vi "Parse GULP Output file.vi"(10 "Reference Energy/atom (pure Crystal) (eV/atom)":dbl=-3.17454527875, 11 "GULP output file":path) -> (0 "Total Lattice Energy (eV)":dbl, 1 "Interfacial Energy (mJ/m²)":dbl, 2 "GB DoF":dbl[](array[numeric]), 3 "Final Structure":T1, 4 "# of atoms":i32, 5 "Data":string[](array[string]))   [LabVIEW 2010]
uses:
  <vilib>/Analysis/NI_AALPro.lvlib
panel:
  out "Lattice vector c":dbl[](array[numeric])
  out "Lattice vector b":dbl[](array[numeric])
  out "Lattice vector a":dbl[](array[numeric])
  out "Grain Boundary Definition":T2={"Grain 1 Orientation"=[1.0, 1.0, 1.0], "Grain 2 Orientation"=[1.0, 1.0, 1.0], "Twist Angle (Deg)"=60.0, "Translation Vector"=[0.0, 0.0, 0.0]}
  out "Headers":string[](array[string])
  out "Initial Structure":T1
  out "GB Area":dbl
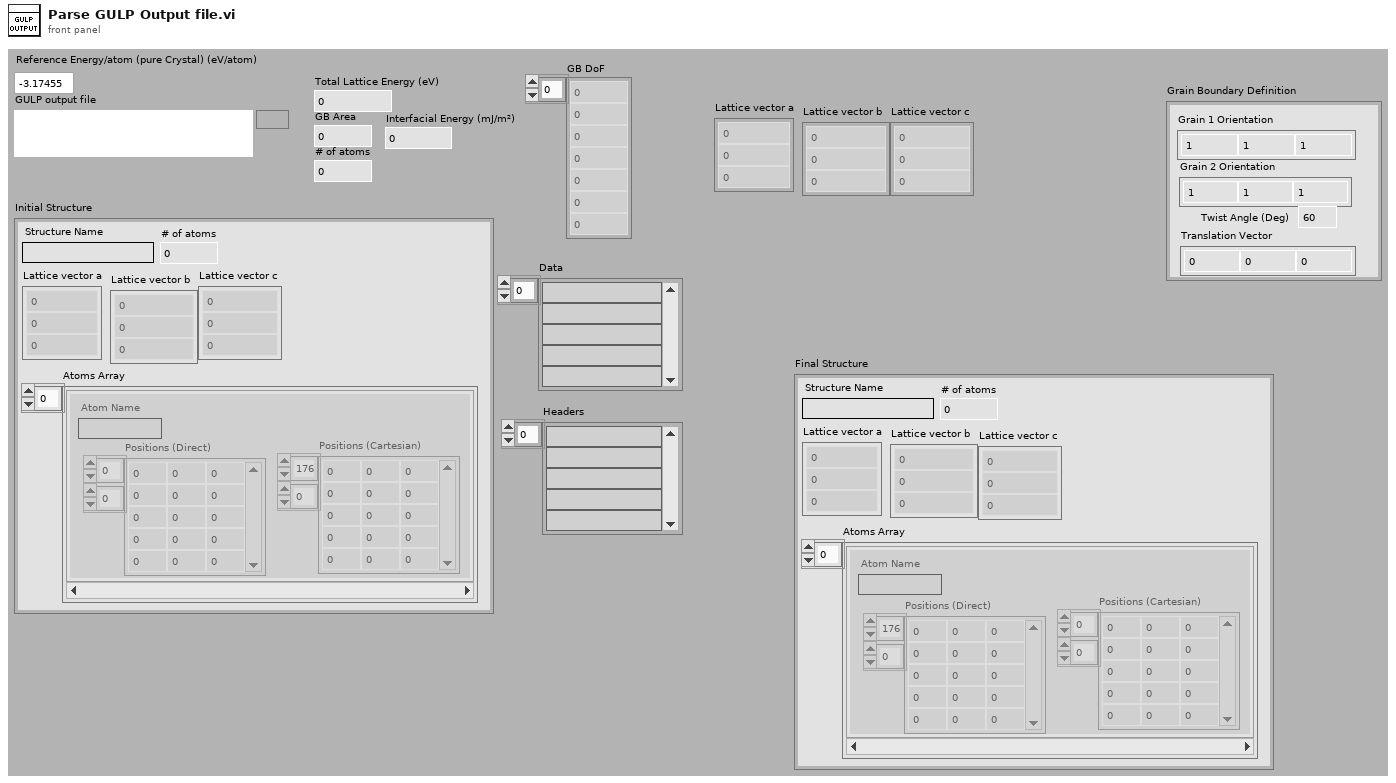
[diagram p1: front panel]
types:
  T1 = cluster{"Structure Name":string, "Lattice vector a":dbl[], "Lattice vector b":dbl[], "Lattice vector c":dbl[], "Atoms Array":cluster{"Atom Name":string, "Positions (Direct)":dbl[][], "Positions (Cartesian)":dbl[][]}[], "# of atoms":i32}
  T2 = cluster{"Grain 1 Orientation":dbl[], "Grain 2 Orientation":dbl[], "Twist Angle (Deg)":dbl, "Translation Vector":dbl[]}
  T3 = cluster{"Atom Name":string, "Positions (Direct)":dbl[][]}[]
  T4 = cluster{"Atom Name":string, "Positions (Direct)":dbl[][]}
  T5 = cluster{"token string":string, "Positions (Direct)":dbl[][]}[]
  T6 = cluster{"Atom Name":string, "Positions (Direct)":dbl[][], dbl[][]}
  T7 = cluster{string, "Lattice vector a":dbl[], "Lattice vector b":dbl[], "Lattice vector c":dbl[], cluster{"Atom Name":string, "Positions (Direct)":dbl[][], dbl[][]}[], "# of atoms":i32}
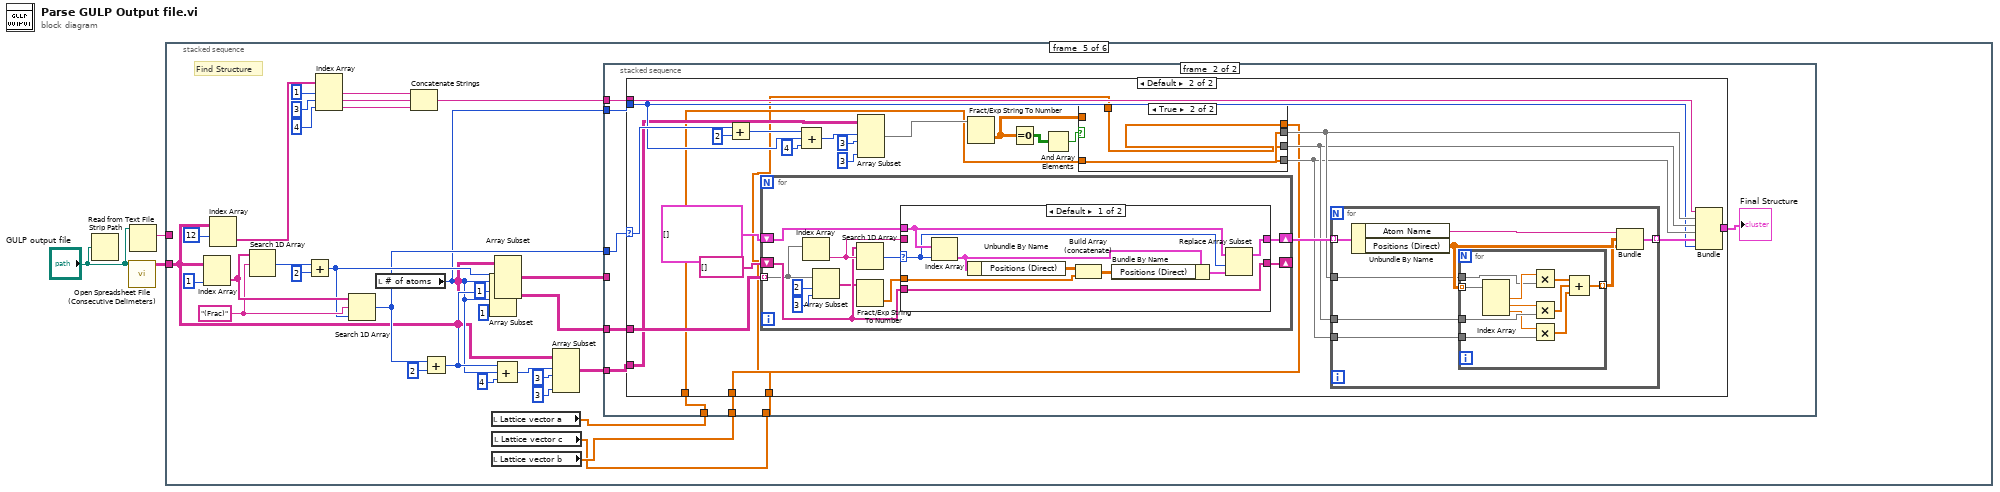
[diagram p0: block diagram]
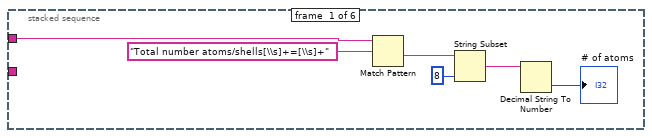
[diagram p2: hidden frame]
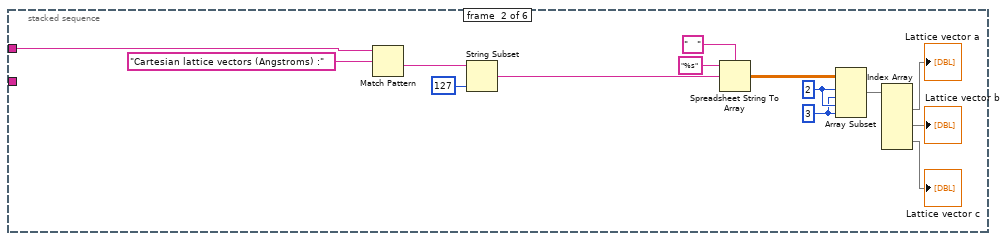
[diagram p3: hidden frame]
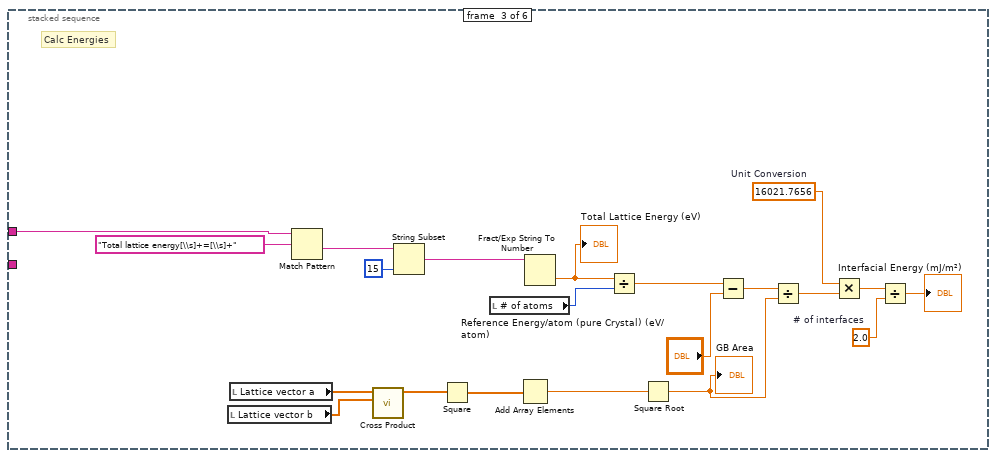
[diagram p4: hidden frame]
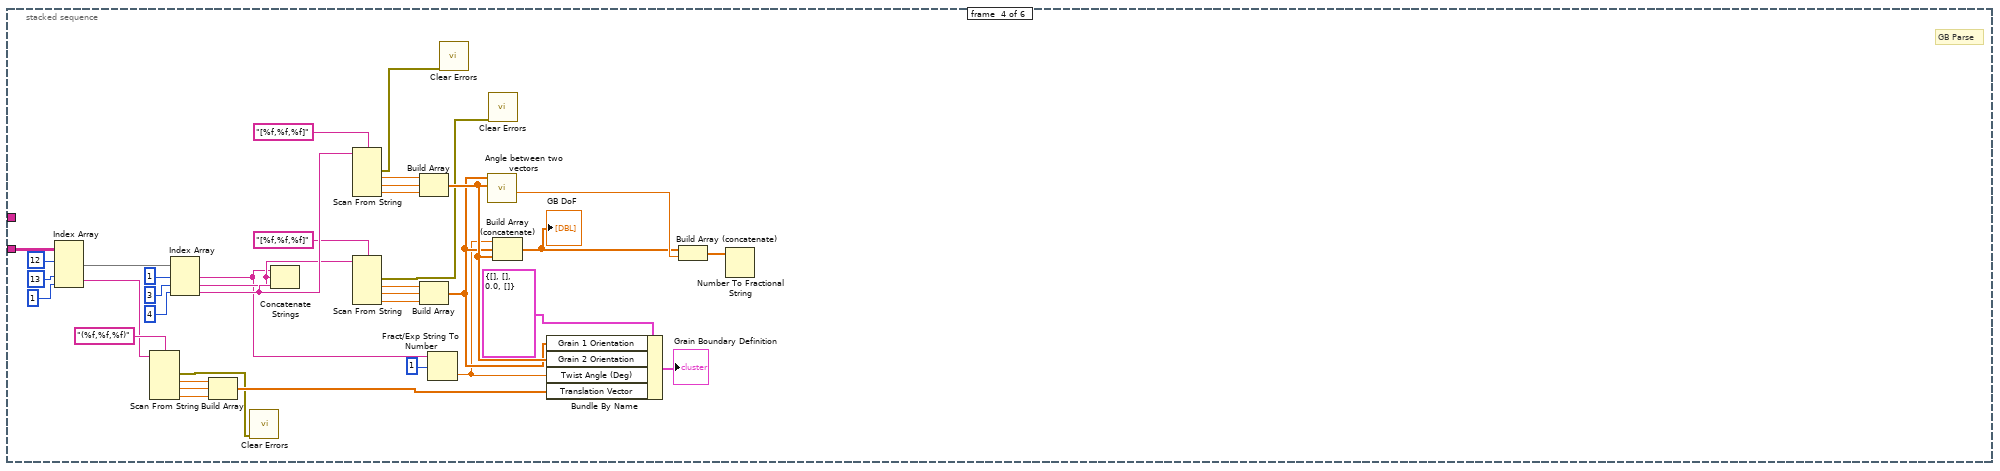
[diagram p5: hidden frame]
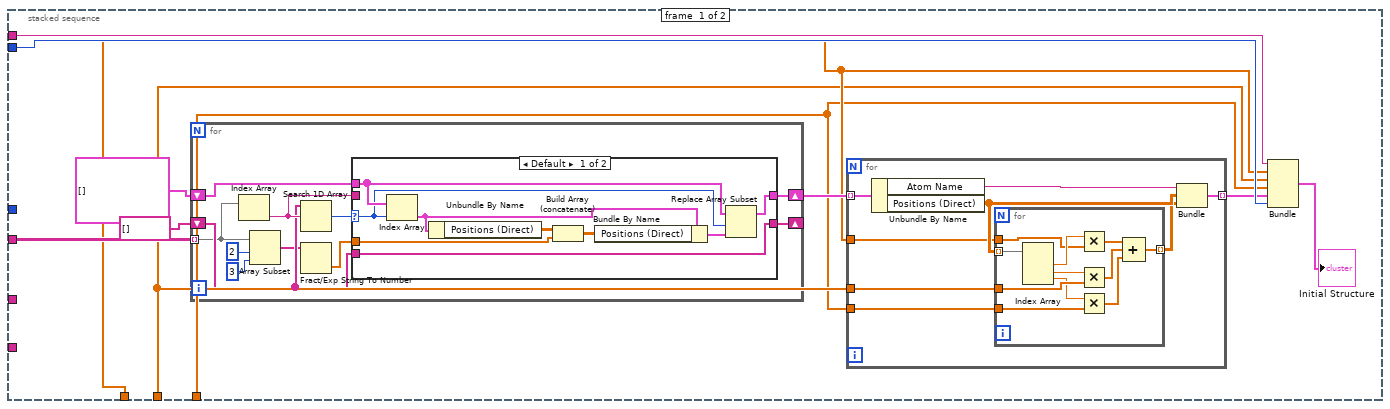
[diagram p6: hidden frame]
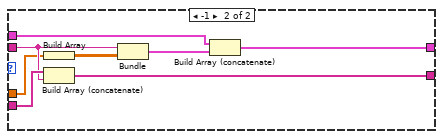
[diagram p7: hidden frame]
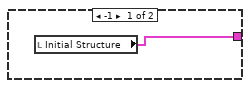
[diagram p8: hidden frame]
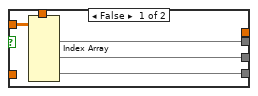
[diagram p9: hidden frame]
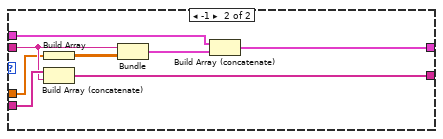
[diagram p10: hidden frame]
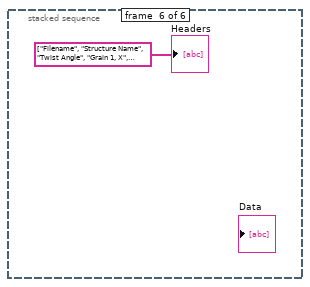
[diagram p11: hidden frame]
diagram:
  n1 = Strip Path(path="GULP output file") -> ()  [unwired: 2 out]
  n2 = call "Open Spreadsheet File (Consecutive Delimeters).vi"("File"="GULP output file") -> ("Array"=w1:string[][])  [unwired: 9 in, 1 out]
  n3 = Read from Text File(file (use dialog)="GULP output file") -> (text=w2:string)  [unwired: 3 in, 3 out]
  n4 = stacked-sequence {
    tunnel: w2 -> [w5 w22 w40 _ _ _]
    tunnel: w1 -> [_ _ _ w51 w84 _]
    frame #0 {
      n5 = Match Pattern(string=w5, regular expression="Total number atoms/shells[\\s]+=[\\s]+") -> (after substring=w7:string)  [unwired: 1 in, 3 out]
      n6 = String Subset(string=w7, length (rest)=8 ("length (rest)")) -> (substring=w9:string)  [unwired: 1 in]
      n7 = Decimal String To Number(string=w9) -> (number=→"# of atoms":i32)  [unwired: 2 in, 1 out]
    }
    frame #1 {
      w15 = 3 ("length")
      w16 = 2 ("index")
      n8 = Match Pattern(string=w22, regular expression="Cartesian lattice vectors (Angstroms) :") -> (after substring=w14:string)  [unwired: 1 in, 3 out]
      n9 = String Subset(string=w14, length (rest)=127 ("length (rest)")) -> (substring=w18:string)  [unwired: 1 in]
      n10 = Spreadsheet String To Array(delimiter (Tab)="   ", format string="%s", spreadsheet string=w18) -> (array=w17:dbl[][])  [unwired: 1 in]
      n11 = Array Subset(array=w17, index (row)=w16, length (row)=w15, index (col)=w16, length (col)=w15) -> (w13:dbl[][])
      n12 = Index Array(array=w13) -> (element #1=→"Lattice vector a":dbl[], element #2=→"Lattice vector b":dbl[], element #3=→"Lattice vector c":dbl[])  [unwired: 6 in]
    }
    frame #2 {
      w35 = 2.0  # # of interfaces
      w34 = 16021.7656  # Unit Conversion
      # "Calc Energies"
      n13 = local read "Lattice vector b"() -> (w29:dbl[])
      n14 = local read "Lattice vector a"() -> (w30:dbl[])
      n15 = Match Pattern(string=w40, regular expression="Total lattice energy[\\s]+=[\\s]+") -> (after substring=w42:string)  [unwired: 1 in, 3 out]
      n16 = call <vilib>:"Cross Product.vi"("B Vector"=w29, "A Vector"=w30) -> ("Cross Product"=w39:dbl[])  [unwired: 8 in, 1 out]
      n17 = String Subset(string=w42, length (rest)=15 ("length (rest)")) -> (substring=w44:string)  [unwired: 1 in]
      n18 = Square(x=w39) -> (x^2=w38:dbl[])
      n19 = local read "# of atoms"() -> (w26:i32)
      n20 = Add Array Elements(numeric array=w38) -> (sum=w37:dbl)
      n21 = Fract/Exp String To Number(string=w44) -> (number=w27:dbl)  [unwired: 3 in, 1 out]
      "Total Lattice Energy (eV)" <- w27
      n22 = Divide(x=w27, y=w26) -> (x/y=w32:dbl)
      n23 = Square Root(x=w37) -> (sqrt(x)=w25:dbl)
      "GB Area" <- w25
      n24 = Subtract(x=w32, y="Reference Energy/atom (pure Crystal) (eV/atom)") -> (x-y=w31:dbl)
      n25 = Divide(x=w31, y=w25) -> (x/y=w33:dbl)
      n26 = Multiply(x=w34, y=w33) -> (x*y=w36:dbl)
      n27 = Divide(x=w36, y=w35) -> (x/y=→"Interfacial Energy (mJ/m²)":dbl)
    }
    frame #3 {
      # "GB Parse"
      n28 = Index Array(array=w51, index (row) #1=12 ("index (row)"), index (row) #2=13 ("index (row)"), index (col) #2=1 ("disabled index (col)")) -> (element #1=w53:string[], element #2=w76:string)  [unwired: 1 in]
      n29 = Scan From String(format string="(%f,%f,%f)", input string=w76) -> (error out=w47:errorcluster, output 1=w78:dbl, output 2=w79:dbl, output 3=w80:dbl)  [unwired: 5 in, 2 out]
      n30 = Index Array(array=w53, index #1=1 ("index"), index #2=3 ("index"), index #3=4 ("index")) -> (element #1=w57:string, element #2=w59:string, element #3=w61:string)
      n31 = Build Array(w78, w79, w80) -> (w81:dbl[])
      n32 = call <vilib>:"Clear Errors.vi"("error in (no error)"=w47) -> ()  [unwired: 6 in, 1 out]
      n33 = Concatenate Strings(w57, w59, w61) -> ()  [unwired: 1 out]
      n34 = Scan From String(format string="[%f,%f,%f]", input string=w61) -> (error out=w46:errorcluster, output 1=w68:dbl, output 2=w69:dbl, output 3=w70:dbl)  [unwired: 5 in, 2 out]
      n35 = Scan From String(format string="[%f,%f,%f]", input string=w59) -> (error out=w45:errorcluster, output 1=w65:dbl, output 2=w66:dbl, output 3=w67:dbl)  [unwired: 5 in, 2 out]
      n36 = Build Array(w68, w69, w70) -> (w73:dbl[])
      n37 = Build Array(w65, w66, w67) -> (w72:dbl[])
      n38 = Fract/Exp String To Number(string=w57, offset=1) -> (number=w49:dbl)  [unwired: 2 in, 1 out]
      n39 = call <vilib>:"Clear Errors.vi"("error in (no error)"=w46) -> ()  [unwired: 6 in, 1 out]
      n40 = call "Angle between two vectors.vi"("Vector 2"=w73, "Vector 1"=w72) -> ("Angle (Degrees)"=w63:dbl)  [unwired: 7 in, 2 out]
      n41 = call <vilib>:"Clear Errors.vi"("error in (no error)"=w45) -> ()  [unwired: 6 in, 1 out]
      n42 = Build Array (concatenate)(w49, w72, w73) -> (w48:dbl[])
      "GB DoF" <- w48
      n43 = Bundle By Name(cluster=T2 {"Grain 1 Orientation"=[], "Grain 2 Orientation"=[], "Twist Angle (Deg)"=0.0, "Translation Vector"=[]} ("Grain Boundary Definition 2"), "Grain 1 Orientation"=w72, "Grain 2 Orientation"=w73, "Twist Angle (Deg)"=w49, "Translation Vector"=w81) -> (→"Grain Boundary Definition":T2)
      n44 = Build Array (concatenate)(w48, w63) -> (w64:dbl[])
      n45 = Number To Fractional String(number=w64) -> ()  [unwired: 3 in, 1 out]
    }
    frame #4 {
      w99 = "(Frac)" ("element")
      # "Find Structure"
      n46 = Index Array(array=w84, index (col)=1 ("disabled index (col)")) -> (element=w100:string[])  [unwired: 1 in]
      n47 = Index Array(array=w84, index (row)=12) -> (element=w82:string[])  [unwired: 1 in]
      n48 = Search 1D Array(1D array=w100, element=w99) -> (index of element=w105:i32)  [unwired: 1 in]
      n49 = Add(x=w105, y=2) -> (x+y=w93:i32)
      n50 = Index Array(array=w82, index #1=1 ("index"), index #2=3 ("index"), index #3=4 ("index")) -> (element #1=w110:string, element #2=w109:string, element #3=w108:string)
      n51 = Search 1D Array(1D array=w100, element=w99, start index (0)=w93) -> (index of element=w89:i32)
      n52 = local read "# of atoms"() -> (w88:i32)
      n53 = Concatenate Strings(w110, w109, w108) -> (w107:string)
      n54 = Add(x=w89, y=2) -> (x+y=w90:i32)
      n55 = Array Subset(array=w84, index (row)=w90, length (row)=w88, index (col)=1 ("index")) -> (w101:string[][])  [unwired: 1 in]
      n56 = local read "Lattice vector a"() -> (w87:dbl[])
      n57 = local read "Lattice vector b"() -> (w86:dbl[])
      n58 = local read "Lattice vector c"() -> (w85:dbl[])
      n59 = Array Subset(array=w84, index (row)=w93, length (row)=w88, index (col)=1 ("index")) -> (w102:string[][])  [unwired: 1 in]
      n60 = Compound Arithmetic op=ADD(w90, w88, 4 ("value")) -> (w91:i32)
      n61 = Array Subset(array=w84, index (row)=w91, length (row)=3 ("length"), length (col)=3 ("length")) -> (w96:string[][])  [unwired: 1 in]
      n62 = stacked-sequence {
        tunnel: w107 -> [w124 w180]
        tunnel: w88 -> [w123 w179]
        tunnel: w102 -> [w121 _]
        tunnel: w101 -> [_ w178]
        tunnel: w96 -> [_ w177]
        tunnel: w89 -> [_ w176]
        tunnel: w87 -> [w117 w174]
        tunnel: w86 -> [w116 w173]
        tunnel: w85 -> [w115 w172]
        frame #0 {
          n63 = for {
            tunnel: w121 -> [w148] mode=indexing
            shift-right: [w152] -> _
            shift-left: string[] [] -> [w151]
            shift-right: [w149] -> w118
            shift-left: T3 [] ("Atoms Array") -> [w150]
            n64 = Index Array(array=w148) -> (element=w153:string)  [unwired: 1 in]
            n65 = Array Subset(array=w148, index=2, length=3) -> (w145:string[])
            n66 = Search 1D Array(1D array=w151, element=w153) -> (index of element=w154:i32)  [unwired: 1 in]
            n67 = Fract/Exp String To Number(string=w145) -> (number=w144:dbl[])  [unwired: 3 in, 1 out]
            n68 = case shown="Default" w154 {
              selector: w154 -> [w157 _]
              tunnel: w153 -> [_ w167]
              tunnel: [w163 w171] -> w152
              tunnel: w151 -> [w163 w170]
              tunnel: w150 -> [w158 w169]
              tunnel: [w155 w168] -> w149
              tunnel: w144 -> [w161 w166]
              frame Default {
                n69 = Index Array(array=w158, index=w157) -> (element=w160:T4)
                n70 = Unbundle By Name(w160) -> ("Positions (Direct)"=w162:dbl[][])
                n71 = Build Array (concatenate)(w162, w161) -> (w159:dbl[][])
                n72 = Bundle By Name(cluster=w160, "Positions (Direct)"=w159) -> (w156:T4)
                n73 = Replace Array Subset(array=w158, new element=w156, index=w157) -> (w155:T3)
              }
              frame -1 {
                n74 = Build Array(w166) -> (w165:dbl[][])
                n75 = Build Array (concatenate)(w170, w167) -> (w171:string[])
                n76 = Bundle("token string"=w167, w165) -> (w164:cluster{"token string":string, dbl[][]})  [unwired: 1 in]
                n77 = Build Array (concatenate)(w169, w164) -> (w168:T5)
              }
            }
          }
          n78 = for {
            tunnel: w118 -> [w132] mode=indexing
            tunnel: w117 -> [w129]
            tunnel: w116 -> [w128]
            tunnel: w115 -> [w127]
            tunnel: [w125] -> w122 mode=indexing
            n79 = Unbundle By Name(w132) -> ("Atom Name"=w131:string, "Positions (Direct)"=w130:dbl[][])
            n80 = for {
              tunnel: w130 -> [w143] mode=indexing
              tunnel: w129 -> [w141]
              tunnel: w128 -> [w139]
              tunnel: w127 -> [w137]
              tunnel: [w133] -> w126 mode=indexing
              n81 = Index Array(array=w143) -> (element #1=w142:dbl, element #2=w140:dbl, element #3=w138:dbl)  [unwired: 3 in]
              n82 = Multiply(x=w142, y=w141) -> (x*y=w136:dbl[])
              n83 = Multiply(x=w140, y=w139) -> (x*y=w135:dbl[])
              n84 = Multiply(x=w138, y=w137) -> (x*y=w134:dbl[])
              n85 = Compound Arithmetic op=ADD(w136, w135, w134) -> (w133:dbl[])
            }
            n86 = Bundle("Atom Name"=w131, "Positions (Direct)"=w130, w126) -> (w125:T6)  [unwired: 1 in]
          }
          n87 = Bundle(w124, "Lattice vector a"=w117, "Lattice vector b"=w116, "Lattice vector c"=w115, w122, "# of atoms"=w123) -> (→"Initial Structure":T7)  [unwired: 1 in]
        }
        frame #1 {
          n88 = case shown="Default" w176 {
            selector: w176 -> [_ w191]
            tunnel: w180 -> [_ w207]
            tunnel: w179 -> [_ w190]
            tunnel: [w181 w205] -> w175
            tunnel: w178 -> [_ w198]
            tunnel: w177 -> [_ w189]
            tunnel: w174 -> [_ w184]
            tunnel: w173 -> [_ w183]
            tunnel: w172 -> [_ w182]
            frame -1 {
              n89 = local read "Initial Structure"() -> (w181:T1)
            }
            frame Default {
              n90 = Add(x=w191, y=2) -> (x+y=w197:i32)
              n91 = for {
                tunnel: w198 -> [w238] mode=indexing
                shift-right: [w242] -> _
                shift-left: string[] [] -> [w241]
                shift-right: [w239] -> w202
                shift-left: T3 [] ("Atoms Array") -> [w240]
                n92 = Index Array(array=w238) -> (element=w243:string)  [unwired: 1 in]
                n93 = Array Subset(array=w238, index=2, length=3) -> (w235:string[])
                n94 = Search 1D Array(1D array=w241, element=w243) -> (index of element=w244:i32)  [unwired: 1 in]
                n95 = Fract/Exp String To Number(string=w235) -> (number=w234:dbl[])  [unwired: 3 in, 1 out]
                n96 = case shown="Default" w244 {
                  selector: w244 -> [w247 _]
                  tunnel: w243 -> [_ w257]
                  tunnel: [w253 w261] -> w242
                  tunnel: w241 -> [w253 w260]
                  tunnel: w240 -> [w248 w259]
                  tunnel: [w245 w258] -> w239
                  tunnel: w234 -> [w251 w256]
                  frame Default {
                    n97 = Index Array(array=w248, index=w247) -> (element=w250:T4)
                    n98 = Unbundle By Name(w250) -> ("Positions (Direct)"=w252:dbl[][])
                    n99 = Build Array (concatenate)(w252, w251) -> (w249:dbl[][])
                    n100 = Bundle By Name(cluster=w250, "Positions (Direct)"=w249) -> (w246:T4)
                    n101 = Replace Array Subset(array=w248, new element=w246, index=w247) -> (w245:T3)
                  }
                  frame -1 {
                    n102 = Build Array(w256) -> (w255:dbl[][])
                    n103 = Build Array (concatenate)(w260, w257) -> (w261:string[])
                    n104 = Bundle("token string"=w257, w255) -> (w254:cluster{"token string":string, dbl[][]})  [unwired: 1 in]
                    n105 = Build Array (concatenate)(w259, w254) -> (w258:T5)
                  }
                }
              }
              n106 = Compound Arithmetic op=ADD(w197, w190, 4 ("value")) -> (w196:i32)
              n107 = Array Subset(array=w189, index (row)=w196, length (row)=3 ("length"), length (col)=3 ("length")) -> (w188:string[][])  [unwired: 1 in]
              n108 = Fract/Exp String To Number(string=w188) -> (number=w187:dbl[][])  [unwired: 3 in, 1 out]
              n109 = Equal To 0?(x=w187) -> (x = 0?=w186:bool[][])
              n110 = And Array Elements(Boolean array=w186) -> (logical AND=w185:bool)
              n111 = case shown="True" w185 {
                tunnel: [w211 w214] -> w201
                tunnel: [w210 w213] -> w200
                tunnel: [w209 w212] -> w199
                tunnel: w187 -> [w208 _]
                tunnel: w184 -> [_ w214]
                tunnel: w183 -> [_ w213]
                tunnel: w182 -> [_ w212]
                frame False {
                  n112 = Index Array(array=w208) -> (element #1=w211:dbl[], element #2=w210:dbl[], element #3=w209:dbl[])  [unwired: 6 in]
                }
                frame True {
                }
              }
              n113 = for {
                tunnel: w202 -> [w222] mode=indexing
                tunnel: w201 -> [w219]
                tunnel: w200 -> [w218]
                tunnel: w199 -> [w217]
                tunnel: [w215] -> w206 mode=indexing
                n114 = Unbundle By Name(w222) -> ("Atom Name"=w221:string, "Positions (Direct)"=w220:dbl[][])
                n115 = for {
                  tunnel: w220 -> [w233] mode=indexing
                  tunnel: w219 -> [w231]
                  tunnel: w218 -> [w229]
                  tunnel: w217 -> [w227]
                  tunnel: [w223] -> w216 mode=indexing
                  n116 = Index Array(array=w233) -> (element #1=w232:dbl, element #2=w230:dbl, element #3=w228:dbl)  [unwired: 3 in]
                  n117 = Multiply(x=w232, y=w231) -> (x*y=w226:dbl[])
                  n118 = Multiply(x=w230, y=w229) -> (x*y=w225:dbl[])
                  n119 = Multiply(x=w228, y=w227) -> (x*y=w224:dbl[])
                  n120 = Compound Arithmetic op=ADD(w226, w225, w224) -> (w223:dbl[])
                }
                n121 = Bundle("Atom Name"=w221, "Positions (Direct)"=w220, w216) -> (w215:T6)  [unwired: 1 in]
              }
              n122 = Bundle(w207, "Lattice vector a"=w201, "Lattice vector b"=w200, "Lattice vector c"=w199, w206, "# of atoms"=w190) -> (w205:T7)  [unwired: 1 in]
            }
          }
          "Final Structure" <- w175
        }
      }
    }
    frame #5 {
      "Headers" <- string[] ["Filename", "Structure Name", "Twist Angle", "Grain 1, X", "Grain 1, Y", "Grain 1, Z", "Grain 2, X", "Grain 2, Y", "Grain 2, Z", "Tilt Angle", "# of atoms", "|A|", "|B|", "|C|", "Total Lattice Energy (eV)", "Interfacial Energy (mJ/m²)"] ("Data 2")
    }
  }
